vi "Using the VI Activation Event for VI Scripting.vi"() -> ()   [LabVIEW 2023]
doc: "This VI demonstrates how to open a reference to other open VIs and perform VI scripting actions on them."
panel:
  out "Active Window":u16(ring) items=["Front Panel", "Block Diagram"]
  out "Selected Object Types":string[](array[string])
  out "Selected VI":string
  in  "Stop":bool
  # "Overview: Demonstrates how to open a reference to other open VIs and perform VI scripting actions on them.\nInstructions:\n1. Open one or more other VIs.\n2. Run this VI.\n3. As you select the panel and diagram window of the other VIs, you should see the Selected VI and Active Window indicators below update.\n4. Select objects on the panels and diagrams of the other VIs. You will see the Selected Object Types list update as you change your selections.\n5. Click Stop to stop the VI."
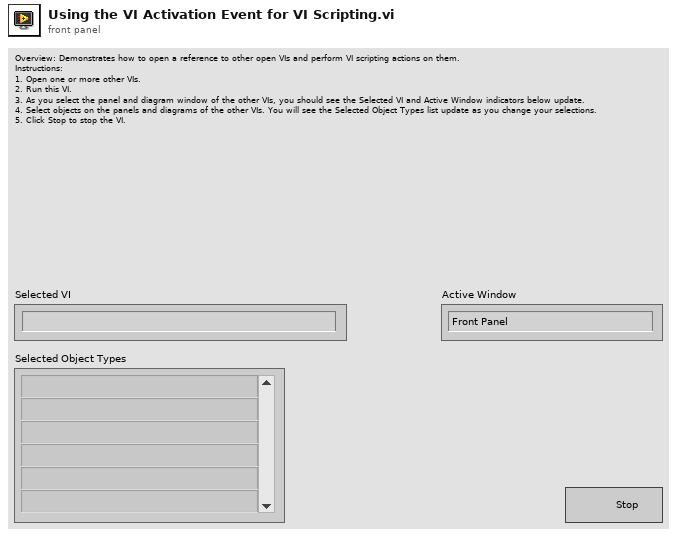
[diagram p1: front panel]
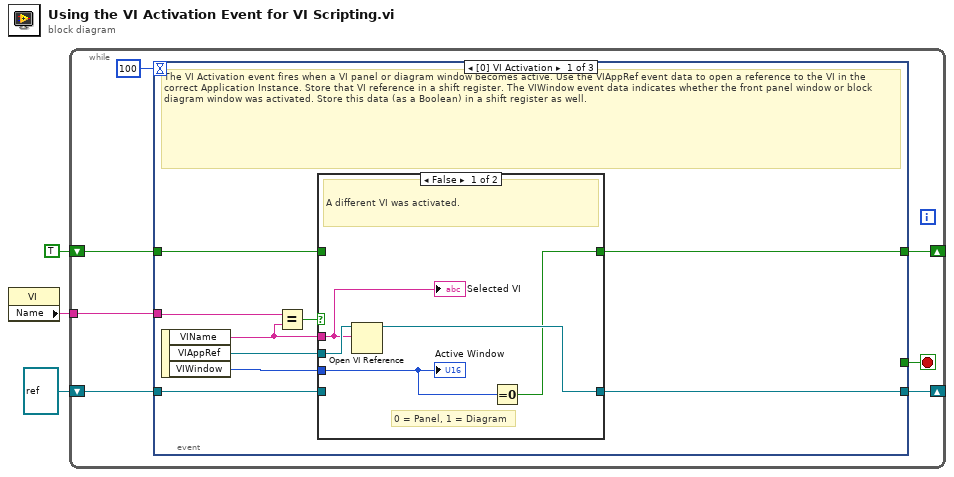
[diagram p0: block diagram]
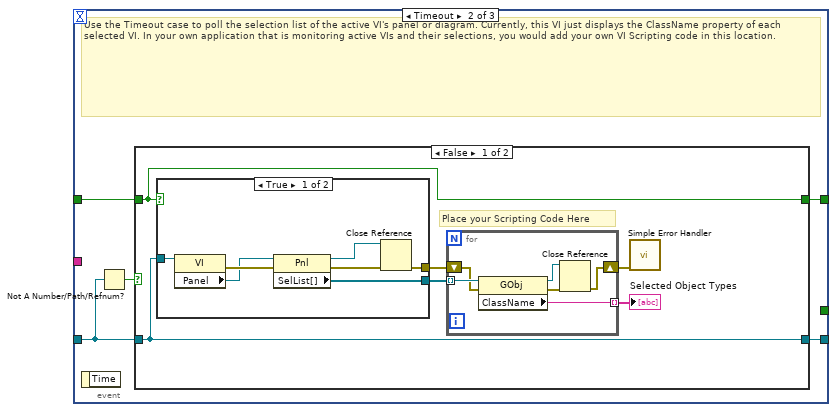
[diagram p3: hidden frame]
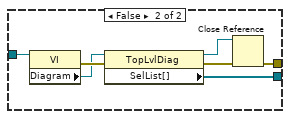
[diagram p4: hidden frame]
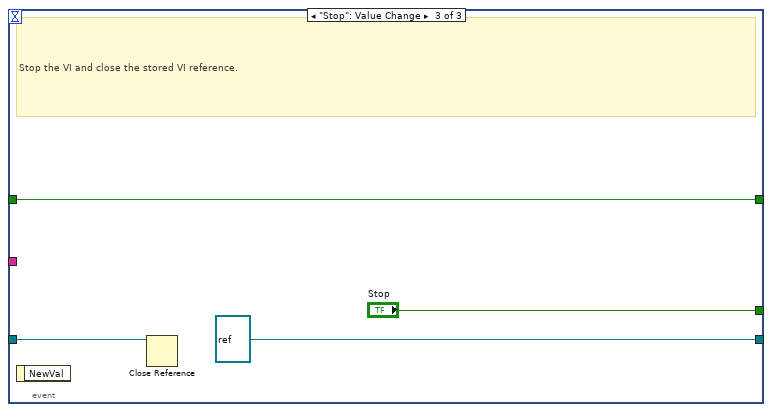
[diagram p6: hidden frame]
diagram:
  n1 = property class="VI"() -> ("Name"=w3:string)  [unwired: 2 in, 2 out]
  n2 = while {
    tunnel: w3 -> [w9]
    shift-right: [w8] -> _
    shift-left: refnum<vi> refnum ("VIAppRef") -> [w7]
    shift-right: [w4] -> _
    shift-left: TRUE -> [w5]
    stop <- w10 stop-if-true
    n3 = event shown="[0] VI Activation" {
      selector: _ -> [_ _ _]
      dyn-events: _ -> [_ _ _]
      timeout: 100 -> [_ _ _]
      tunnel: [_ _ "Stop"] -> w10
      tunnel: w9 -> [w18 _ _]
      tunnel: [w14 w30 refnum<vi> refnum ("VIAppRef")] -> w8
      tunnel: w7 -> [w17 w29 w61]
      tunnel: w5 -> [w12 w28 w62]
      tunnel: [w11 w27 w62] -> w4
      event VI Activation {
        # "The VI Activation event fires when a VI panel or diagram window becomes active. Use the VIAppRef event data to open a reference to the VI in the correct Application Instance. Store that VI reference in a shift register. The VIWindow event data indicates whether the front panel window or block diagram window was activated. Store this data (as a Boolean) in a shift register as well."
        n4 = event-data() -> ("VIName"=w15:string, "VIAppRef"=w16:refnum<vi>, "VIWindow"=w13:i32)  [unwired: 1 out]
        n5 = Equal?(x=w18, y=w15) -> (x = y?=w19:bool)
        n6 = case shown="False" w19 {
          tunnel: [w21 w26] -> w14
          tunnel: w17 -> [_ w26]
          tunnel: w15 -> [w23 _]
          tunnel: w16 -> [w24 _]
          tunnel: w13 -> [w22 _]
          tunnel: w12 -> [_ w25]
          tunnel: [w20 w25] -> w11
          frame False {
            # "0 = Panel, 1 = Diagram"
            # "A different VI was activated."
            n7 = Open VI Reference(application reference (local)=w24, vi path=w23) -> (vi reference=w21:refnum<vi>)  [unwired: 4 in, 1 out]
            n8 = Equal To 0?(x=w22) -> (x = 0?=w20:bool)
            "Selected VI" <- w23
            "Active Window" <- w22
          }
          frame True {
            # "This VI was activated. Ignore the activation."
          }
        }
      }
      event Timeout {
        # "Use the Timeout case to poll the selection list of the active VI's panel or diagram. Currently, this VI just displays the ClassName property of each selected VI. In your own application that is monitoring active VIs and their selections, you would add your own VI Scripting code in this location."
        n9 = event-data() -> ()  [unwired: 2 out]
        n10 = Not A Number/Path/Refnum?(number/path/refnum=w29) -> (NaN/Path/Refnum?=w31:bool)
        n11 = case shown="False" w31 {
          tunnel: w28 -> [w33 w58]
          tunnel: w29 -> [w32 w59]
          tunnel: [w32 w59] -> w30
          tunnel: [w33 w58] -> w27
          frame False {
            # "Place your Scripting Code Here"
            n12 = case shown="True" w33 {
              tunnel: [w48 w56] -> w37
              tunnel: [w46 w54] -> w36
              tunnel: w32 -> [w44 w52]
              frame True {
                n13 = property class="VI"(reference=w44) -> (error out=w50:errorcluster, "Panel"=w49:refnum<vi>)  [unwired: 1 in, 1 out]
                n14 = property class="Pnl"(reference=w49, error in=w50) -> (reference out=w45:refnum<vi>, error out=w47:errorcluster, "SelList[]"=w48:refnum<vi>[])
                n15 = Close Reference(reference=w45, error in (no error)=w47) -> (error out=w46:errorcluster)
              }
              frame False {
                n16 = property class="VI"(reference=w52) -> (error out=w57:errorcluster, "Diagram"=w51:refnum<vi>)  [unwired: 1 in, 1 out]
                n17 = property class="TopLvlDiag"(reference=w51, error in=w57) -> (reference out=w53:refnum<vi>, error out=w55:errorcluster, "SelList[]"=w56:refnum<vi>[])
                n18 = Close Reference(reference=w53, error in (no error)=w55) -> (error out=w54:errorcluster)
              }
            }
            n19 = for {
              tunnel: w37 -> [w43] mode=indexing
              tunnel: [w41] -> w35 mode=indexing
              shift-right: [w39] -> w34
              shift-left: w36 -> [w42]
              n20 = property class="GObj"(reference=w43, error in=w42) -> (reference out=w38:refnum<vi>, error out=w40:errorcluster, "ClassName"=w41:string)
              n21 = Close Reference(reference=w38, error in (no error)=w40) -> (error out=w39:errorcluster)
            }
            "Selected Object Types" <- w35
            n22 = call <vilib>:"Simple Error Handler.vi"("error in (no error)"=w34) -> ()  [unwired: 4 in, 5 out]
          }
          frame True {
          }
        }
      }
      event "Stop": Value Change {
        # "Stop the VI and close the stored VI reference."
        n23 = event-data() -> ()  [unwired: 2 out]
        n24 = Close Reference(reference=w61) -> ()  [unwired: 1 in, 1 out]
      }
    }
  }
